vi "Auto Loop 2.vi"(2 "Auto State":u8, 3 "Call Context":T3) -> (0 "Loop 2 Data":T1, 1 "SubState 2":T2)   [LabVIEW 2013]
uses:
  <vilib>/Rock Robotics/WPI/DriverStation/WPI_DriverStationDerivedRobotMode.ctl
  typedefs/State Machine/subStates.ctl
  typedefs/Loop Datatypes/Loop 2 Datatype.ctl
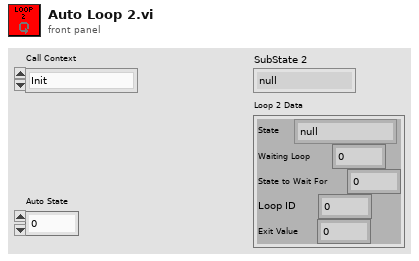
[diagram p1: front panel]
types:
  T1 = typedef "Loop 2 Datatype.ctl" = cluster{"State":T2, "Waiting Loop":i32, "State to Wait For":i32, "Loop ID":i32, "Exit Value":i32}
  T2 = typedef "subStates.ctl" = enum16{"null", "wait", "driver control", "auto", "manual override", "hold position", "rotate", "test", "end"}
  T3 = typedef "WPI_DriverStationDerivedRobotMode.ctl" = enum16{"Init", "Execute", "Stop"}
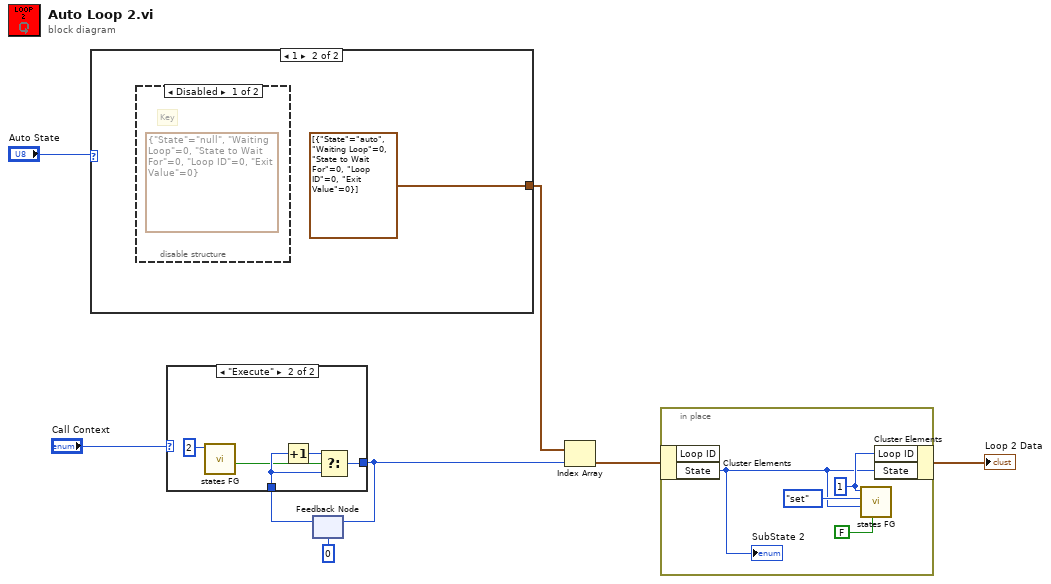
[diagram p0: block diagram]
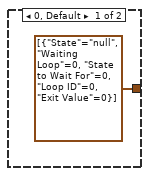
[diagram p2: hidden frame]
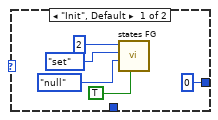
[diagram p4: hidden frame]
diagram:
  n1 = case shown="1" "Auto State" {
    tunnel: [T1[] [{"State"=enum."null", "Waiting Loop"=0, "State to Wait For"=0, "Loop ID"=0, "Exit Value"=0}] T1[] [{"State"=enum."auto", "Waiting Loop"=0, "State to Wait For"=0, "Loop ID"=0, "Exit Value"=0}]] -> w5
    frame 0, Default {
    }
    frame 1 {
      n2 = disable-structure shown="Disabled" {
        frame Disabled {
          (unwired) T1 {"State"=enum."null", "Waiting Loop"=0, "State to Wait For"=0, "Loop ID"=0, "Exit Value"=0} ("Loop 2 Data")
          # "Key"
        }
        frame Enabled {
        }
      }
    }
  }
  n3 = feedback #1(0) -> (w6:i32)
  n4 = case shown="\"Execute\"" "Call Context" {
    tunnel: w6 -> [_ w20]
    tunnel: [0 w18] -> w4
    frame "Init", Default {
      n5 = call "states FG.vi"("exit in"=TRUE, "subState in"=subStates."null", "menu (get)"=enum16{"set", "get"}."set", "Loop ID"=2) -> ()  [unwired: 4 in, 4 out]
    }
    frame "Execute" {
      n6 = call "states FG.vi"("Loop ID"=2) -> ("exit out"=w17:bool)  [unwired: 7 in, 3 out]
      n7 = Increment(x=w20) -> (x+1=w16:i32)
      n8 = Select(t=w16, s=w17, f=w20) -> (s? t:f=w18:i32)
    }
  }
  n9 = feedback-in #1(w4) -> ()
  n10 = Index Array(array=w5, index=w4) -> (element=w2:T1)
  n11 = in-place {
    w22 = 1 ("Loop ID")
    n12 = in-place-cluster #2(w2) -> ("State"=w21:T2)  [unwired: 1 out]
    "SubState 2" <- w21
    n13 = call "states FG.vi"("exit in"=FALSE, "subState in"=w21, "menu (get)"=enum16{"set", "get"}."set", "Loop ID"=w22) -> ()  [unwired: 4 in, 4 out]
    n14 = in-place-cluster #2("Loop ID"=w22, "State"=w21) -> (→"Loop 2 Data":T1)
  }
